vi "GlobalStat to DBLs.vi"(10 "port index":i32, 11 "GlobalStat in":T1) -> (3 "GlobalStat DBL Array":dbl[](array[numeric]))   [LabVIEW 2020, in "AIM ARINC 664 Engine.lvlib" / "Implementation.lvlib" / "Monitor Execution Unit.lvclass"]
doc: "Converts a GlobalStat cluster into a table."
uses:
  Monitor Execution Unit.lvclass
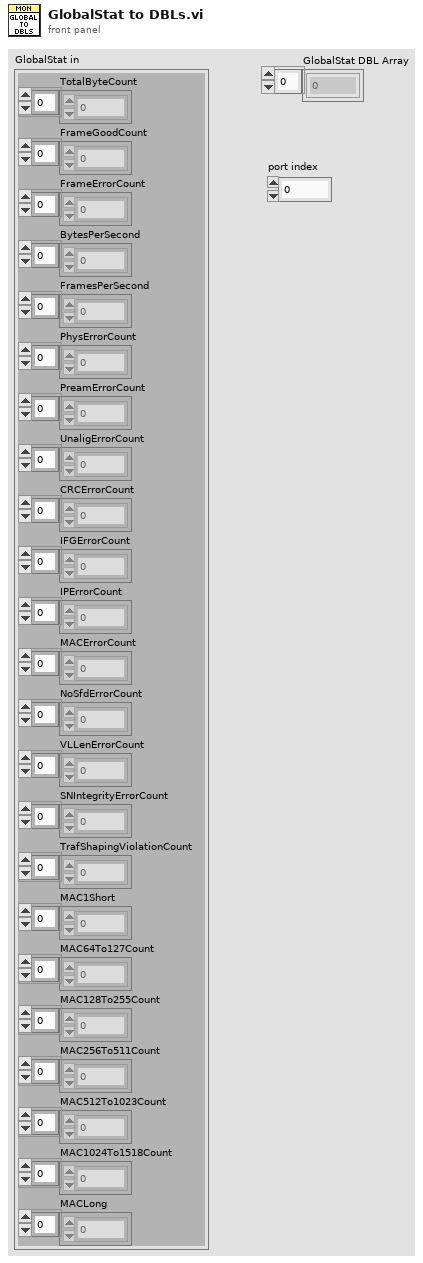
[diagram p1: front panel]
types:
  T1 = cluster{"TotalByteCount":u32[], "FrameGoodCount":u32[], "FrameErrorCount":u32[], "BytesPerSecond":u32[], "FramesPerSecond":u32[], "PhysErrorCount":u32[], "PreamErrorCount":u32[], "UnaligErrorCount":u32[], "CRCErrorCount":u32[], "IFGErrorCount":u32[], "IPErrorCount":u32[], "MACErrorCount":u32[], "NoSfdErrorCount":u32[], "VLLenErrorCount":u32[], "SNIntegrityErrorCount":u32[], "TrafShapingViolationCount":u32[], "MAC1Short":u32[], "MAC64To127Count":u32[], "MAC128To255Count":u32[], "MAC256To511Count":u32[], "MAC512To1023Count":u32[], "MAC1024To1518Count":u32[], "MACLong":u32[]}
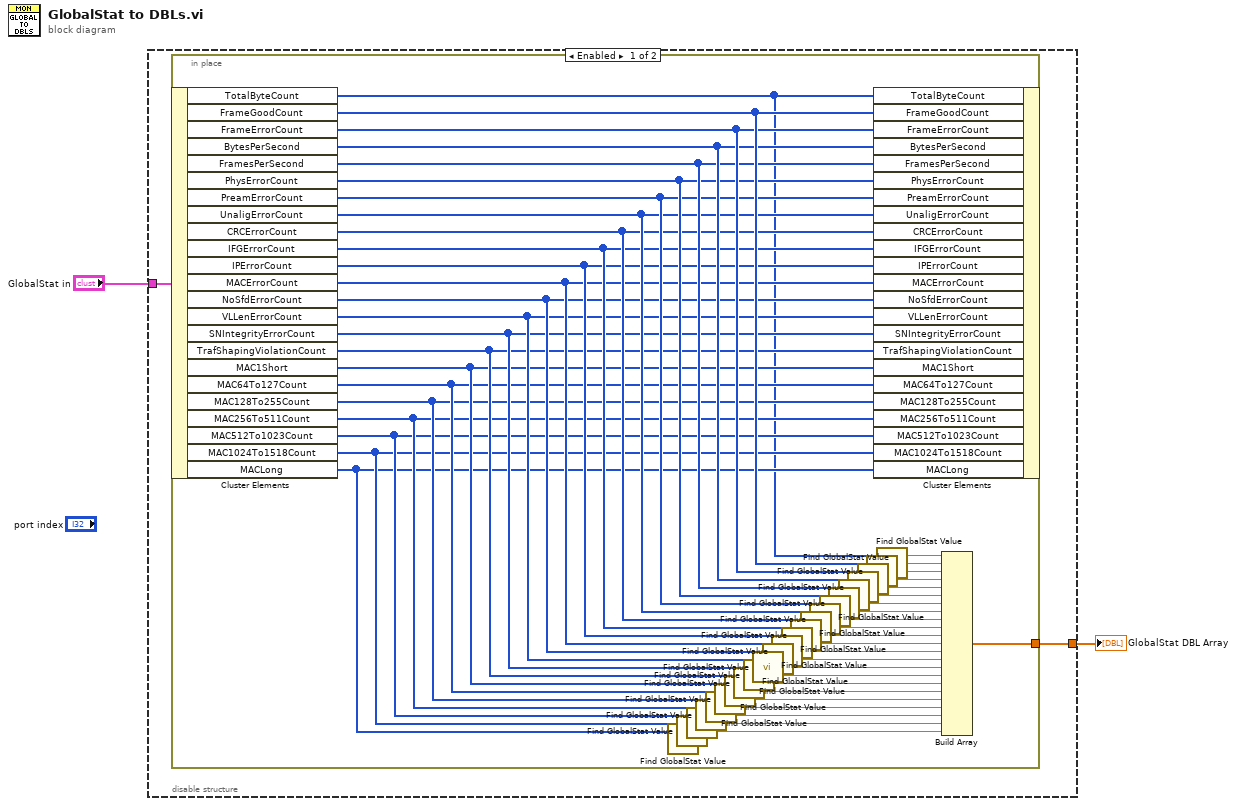
[diagram p0: block diagram]
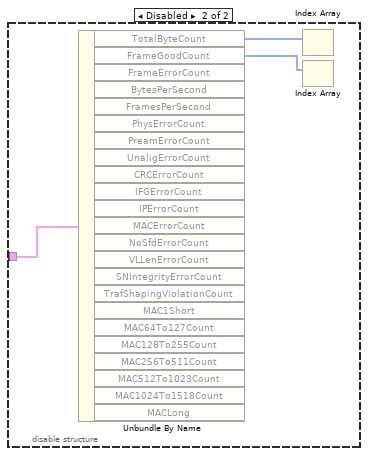
[diagram p2: hidden frame]
diagram:
  n1 = disable-structure shown="Enabled" {
    disable-tunnel: "GlobalStat in" -> [w4 w54]
    disable-tunnel: [w3 _] -> w1
    frame Enabled {
      n2 = in-place {
        in-place-border: [w28] -> w3
        n3 = in-place-cluster #1(w4) -> ("TotalByteCount"=w5:u32[], "FrameGoodCount"=w27:u32[], "FrameErrorCount"=w26:u32[], "BytesPerSecond"=w25:u32[], "FramesPerSecond"=w24:u32[], "PhysErrorCount"=w23:u32[], "PreamErrorCount"=w22:u32[], "UnaligErrorCount"=w21:u32[], "CRCErrorCount"=w20:u32[], "IFGErrorCount"=w19:u32[], "IPErrorCount"=w18:u32[], "MACErrorCount"=w17:u32[], "NoSfdErrorCount"=w16:u32[], "VLLenErrorCount"=w15:u32[], "SNIntegrityErrorCount"=w14:u32[], "TrafShapingViolationCount"=w13:u32[], "MAC1Short"=w12:u32[], "MAC64To127Count"=w11:u32[], "MAC128To255Count"=w10:u32[], "MAC256To511Count"=w9:u32[], "MAC512To1023Count"=w8:u32[], "MAC1024To1518Count"=w7:u32[], "MACLong"=w6:u32[])
        n4 = call "Find GlobalStat Value.vi"("Array"=w6) -> ("GlobalStat value"=w39:dbl)  [unwired: 2 in]
        n5 = call "Find GlobalStat Value.vi"("Array"=w7) -> ("GlobalStat value"=w40:dbl)  [unwired: 2 in]
        n6 = call "Find GlobalStat Value.vi"("Array"=w8) -> ("GlobalStat value"=w41:dbl)  [unwired: 2 in]
        n7 = call "Find GlobalStat Value.vi"("Array"=w9) -> ("GlobalStat value"=w44:dbl)  [unwired: 2 in]
        n8 = call "Find GlobalStat Value.vi"("Array"=w10) -> ("GlobalStat value"=w45:dbl)  [unwired: 2 in]
        n9 = call "Find GlobalStat Value.vi"("Array"=w11) -> ("GlobalStat value"=w46:dbl)  [unwired: 2 in]
        n10 = call "Find GlobalStat Value.vi"("Array"=w12) -> ("GlobalStat value"=w47:dbl)  [unwired: 2 in]
        n11 = call "Find GlobalStat Value.vi"("Array"=w13) -> ("GlobalStat value"=w49:dbl)  [unwired: 2 in]
        n12 = call "Find GlobalStat Value.vi"("Array"=w14) -> ("GlobalStat value"=w50:dbl)  [unwired: 2 in]
        n13 = call "Find GlobalStat Value.vi"("Array"=w15) -> ("GlobalStat value"=w51:dbl)  [unwired: 2 in]
        n14 = call "Find GlobalStat Value.vi"("Array"=w16) -> ("GlobalStat value"=w48:dbl)  [unwired: 2 in]
        n15 = call "Find GlobalStat Value.vi"("Array"=w17) -> ("GlobalStat value"=w43:dbl)  [unwired: 2 in]
        n16 = call "Find GlobalStat Value.vi"("Array"=w18) -> ("GlobalStat value"=w42:dbl)  [unwired: 2 in]
        n17 = call "Find GlobalStat Value.vi"("Array"=w19) -> ("GlobalStat value"=w38:dbl)  [unwired: 2 in]
        n18 = call "Find GlobalStat Value.vi"("Array"=w20) -> ("GlobalStat value"=w37:dbl)  [unwired: 2 in]
        n19 = call "Find GlobalStat Value.vi"("Array"=w21) -> ("GlobalStat value"=w36:dbl)  [unwired: 2 in]
        n20 = call "Find GlobalStat Value.vi"("Array"=w22) -> ("GlobalStat value"=w35:dbl)  [unwired: 2 in]
        n21 = call "Find GlobalStat Value.vi"("Array"=w23) -> ("GlobalStat value"=w34:dbl)  [unwired: 2 in]
        n22 = call "Find GlobalStat Value.vi"("Array"=w24) -> ("GlobalStat value"=w33:dbl)  [unwired: 2 in]
        n23 = call "Find GlobalStat Value.vi"("Array"=w25) -> ("GlobalStat value"=w32:dbl)  [unwired: 2 in]
        n24 = call "Find GlobalStat Value.vi"("Array"=w26) -> ("GlobalStat value"=w31:dbl)  [unwired: 2 in]
        n25 = call "Find GlobalStat Value.vi"("Array"=w27) -> ("GlobalStat value"=w30:dbl)  [unwired: 2 in]
        n26 = in-place-cluster #1("TotalByteCount"=w5, "FrameGoodCount"=w27, "FrameErrorCount"=w26, "BytesPerSecond"=w25, "FramesPerSecond"=w24, "PhysErrorCount"=w23, "PreamErrorCount"=w22, "UnaligErrorCount"=w21, "CRCErrorCount"=w20, "IFGErrorCount"=w19, "IPErrorCount"=w18, "MACErrorCount"=w17, "NoSfdErrorCount"=w16, "VLLenErrorCount"=w15, "SNIntegrityErrorCount"=w14, "TrafShapingViolationCount"=w13, "MAC1Short"=w12, "MAC64To127Count"=w11, "MAC128To255Count"=w10, "MAC256To511Count"=w9, "MAC512To1023Count"=w8, "MAC1024To1518Count"=w7, "MACLong"=w6) -> ()  [unwired: 1 out]
        n27 = call "Find GlobalStat Value.vi"("Array"=w5) -> ("GlobalStat value"=w29:dbl)  [unwired: 2 in]
        n28 = Build Array(w29, w30, w31, w32, w33, w34, w35, w36, w37, w38, w42, w43, w48, w51, w50, w49, w47, w46, w45, w44, w41, w40, w39) -> (w28:dbl[])
      }
    }
    frame Disabled {
      n29 = Unbundle By Name(w54) -> ("TotalByteCount"=w53:u32[], "FrameGoodCount"=w52:u32[])  [unwired: 21 out]
      n30 = Index Array(array=w53) -> ()  [unwired: 1 in, 1 out]
      n31 = Index Array(array=w52) -> ()  [unwired: 1 in, 1 out]
    }
  }
  "GlobalStat DBL Array" <- w1
